vi "DSF.Engine.Sequencer.Get Transfer Group Timings.vi"(8 "error in (no error)":errorcluster, 11 "Sequencer Bundle in":refnum<class "Sequencer Bundle.lvclass">) -> (0 "error out":errorcluster, 2 "Transfer Group Timings":refnum<class "DSF.Engine.Timing.lvclass">[](array[class]), 3 "Sequencer Bundle out":refnum<class "Sequencer Bundle.lvclass">)   [LabVIEW 2016, in "DSF.Engine.lvlib" / "Sequencer Bundle.lvclass"]
uses:
  Sequencer Bundle.lvclass
  Timing/DSF.Engine.Timing.lvclass
  Sequencer Bundle.lvclass/Sequencer Bundle.ctl
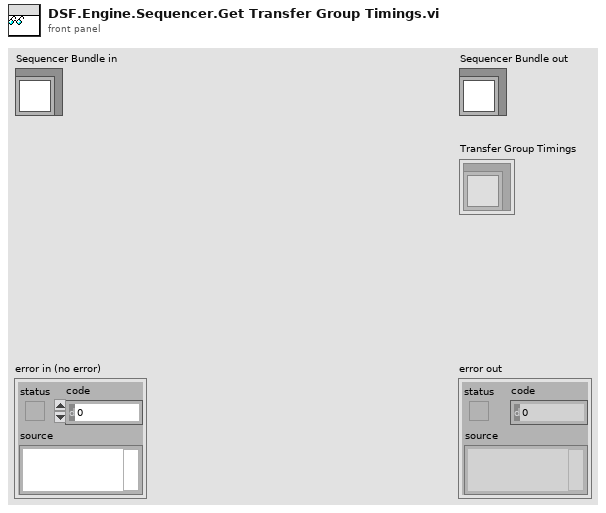
[diagram p1: front panel]
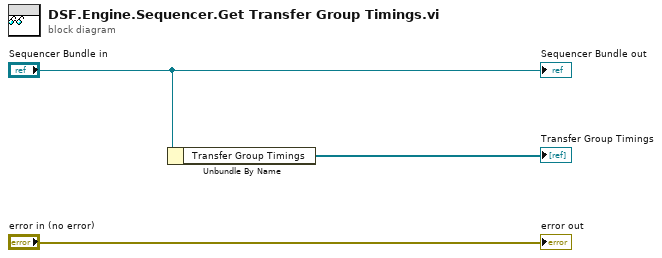
[diagram p0: block diagram]
diagram:
  n1 = Unbundle By Name("Sequencer Bundle in") -> ("Transfer Group Timings"=→"Transfer Group Timings":refnum<class "DSF.Engine.Timing.lvclass">[])
  "error out" <- "error in (no error)"
  "Sequencer Bundle out" <- "Sequencer Bundle in"
